vi "GSIOCBuffered.vi"(4 "Timeout (ms)":i32=2000, 5 "Max":i32=20, 6 "Command":string, 7 "ID":i32) -> (2 "Response":string, 3 "ID out":i32)   [LabVIEW 2012]
uses:
  Gsioc32.dll
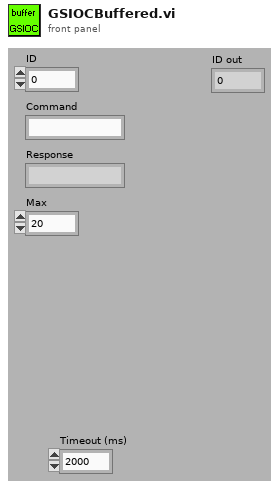
[diagram p1: front panel]
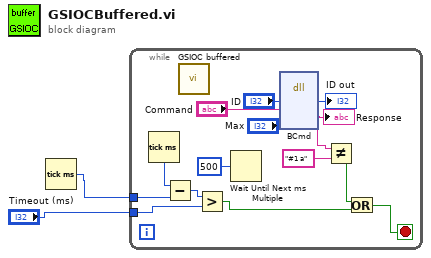
[diagram p0: block diagram]
diagram:
  n1 = Tick Count (ms)() -> (millisecond timer value=w2:u32)
  n2 = while {
    tunnel: w2 -> [w8]
    tunnel: "Timeout (ms)" -> [w7]
    stop <- w4 stop-if-true
    n3 = Tick Count (ms)() -> (millisecond timer value=w9:u32)
    n4 = Subtract(x=w9, y=w8) -> (x-y=w10:u32)
    n5 = call "GSIOC buffered.vi"() -> ()  [unwired: 9 in, 3 out]
    n6 = Greater?(x=w10, y=w7) -> (0:w5:bool)
    n7 = Wait Until Next ms Multiple(millisecond multiple=u32 500) -> ()  [unwired: 1 out]
    n8 = dll-call lib="C:/Users/mw24/Documents/LabVIEW Code 2013 - Fleetwood/Rapid Filter Tester 2/Gsioc32.dll" fn="BCmd"("ID"="ID", "Cmd"="Command", "Max"="Max") -> ("ID"=→"ID out":i32, "Rsp"=w11:string)  [unwired: 7 in, 2 out]
    "Response" <- w11
    n9 = Not Equal?(x=w11, y="#1 a") -> (x != y?=w6:bool)
    n10 = Or(x=w6, y=w5) -> (x .or. y?=w4:bool)
  }
